vi "Example - Call endpoint with MessagePack.vi"() -> ()   [LabVIEW 2020, in "wamplv.lvlib"]
uses:
  wamplv.lvlib
  WAMP Client/API/TypeDefs/Serialisation.ctl
  WAMP Client/WAMP Client.lvclass/WAMP Client.ctl
  Private/Requests/CallRequest (MsgPack)/CallRequest (MsgPack).lvclass/CallRequest (MsgPack).ctl
  WAMP Client/API/WAMP/MsgPack/Call (async) MsgPack.vi
  WAMP Client/Private/SubVIs/Raise Internal Message.vi
  WAMP Client/API/WAMP/MsgPack/Call (async) MsgPack.vi/44dd0fb6-e4b1-424e-8704-d5c62803e1d5.vi
  Private/Requests/CallRequest (MsgPack)/Write Call request.vi
  WAMP Client/Private/SubVIs/Can send requests.vi
  WAMP Client/API/Is Connected.vi
  WAMP Client/Private/SubVIs/Matches serialisation type.vi
  <vilib>/Utility/error.llb/Error Cluster From Error Code.vi
  WAMP Client/Private/SubVIs/Check URI.vi
  MessagePack/MsgPackMap/MsgPackMap.lvclass
  MessagePack/MsgPackArray/MsgPackArray.lvclass
  Private/Requests/CallRequest (MsgPack)/CallRequest (MsgPack).lvclass
  WAMP Client/WAMP Client.lvclass
panel:
  in  "Endpoint URI":string="test.topic"
  in  "Realm":string="default_realm"
  in  "Router URL":string="ws://localhost:8080/"
  # "Example: call endpoint with messagepack"
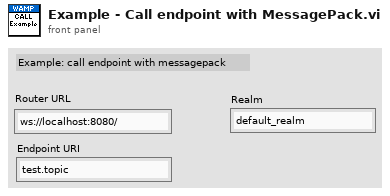
[diagram p1: front panel]
types:
  T1 = typedef "wamplv.lvlib/WAMP Client.lvclass/Serialisation.ctl" = enum16{"JSON", "MessagePack"}
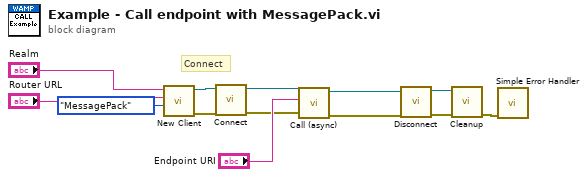
[diagram p0: block diagram]
diagram:
  # "Connect"
  n1 = call "New Client.vi"("Serialisation"=Serialisation."MessagePack", "Address"="Router URL", "Realm"="Realm") -> ("error out"=w8:errorcluster, "WAMP client out"=w11:refnum<class "WAMP Client.lvclass">)  [unwired: 7 in]
  n2 = call "Connect.vi"("error in"=w8, "WAMP Client in"=w11) -> ("error out"=w3:errorcluster, "WAMP Client out"=w5:refnum<class "WAMP Client.lvclass">)  [unwired: 8 in]
  n3 = call-poly "Call (async).vi"("error in (no error)"=w3, "Topic URI"="Endpoint URI", "WAMP Client in"=w5) -> ("error out"=w1:errorcluster, "WAMP Client out"=w2:refnum<class "WAMP Client.lvclass">)  [unwired: 6 in, 1 out]
  n4 = call-dynamic "Disconnect.vi"("error in"=w1, "WAMP Client in"=w2) -> ("error out"=w7:errorcluster, "WAMP Client out"=w10:refnum<class "WAMP Client.lvclass">)  [unwired: 8 in]
  n5 = call-dynamic "Cleanup.vi"("error in"=w7, "WAMP Client in"=w10) -> ("error out"=w9:errorcluster)  [unwired: 8 in, 1 out]
  n6 = call <vilib>:"Simple Error Handler.vi"("error in (no error)"=w9) -> ()  [unwired: 4 in, 5 out]
